vi "利用74HC74设计2-4分频器.vi"() -> ()   [LabVIEW 2018]
panel:
  in  "结束":bool
  out "Q2":bool
  out "Q1":bool
  in  "cp":bool
  # "74HC74：双上升沿D触发器"
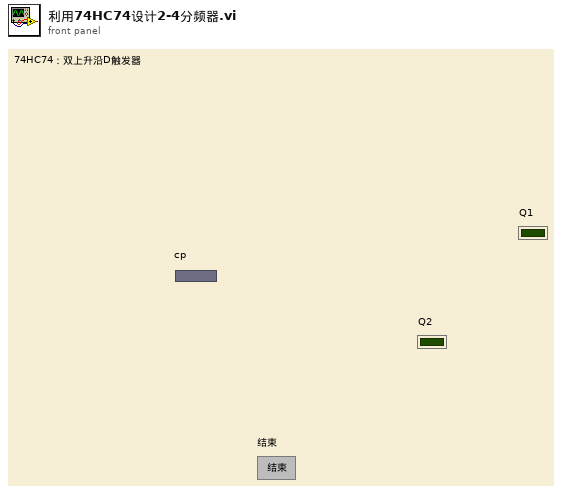
[diagram p1: front panel]
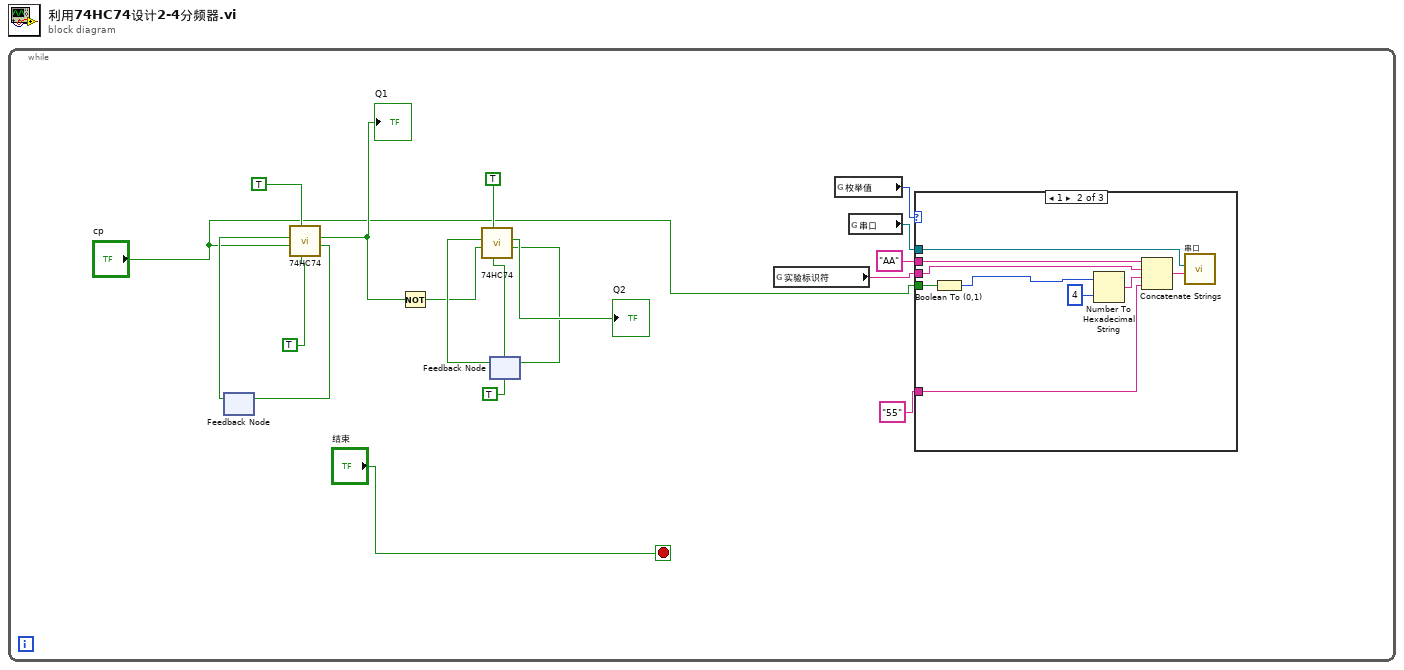
[diagram p0: block diagram]
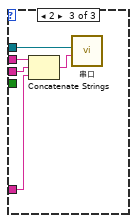
[diagram p3: hidden frame]
diagram:
  n1 = while {
    stop <- "结束" stop-if-true
    n2 = feedback #1() -> (w15:bool)  [unwired: 1 in]
    n3 = call "74HC74.vi"("R`"=TRUE, "S`"=TRUE, "cp"="cp", "D"=w15) -> ("Q`"=w16:bool, "Q"=w8:bool)  [unwired: 6 in]
    "Q1" <- w8
    n4 = feedback-in #1(w16) -> ()
    n5 = Not(x=w8) -> (.not. x?=w9:bool)
    n6 = feedback #2() -> (w10:bool)  [unwired: 1 in]
    n7 = call "74HC74.vi"("R`"=TRUE, "S`"=TRUE, "cp"=w9, "D"=w10) -> ("Q`"=w11:bool, "Q"=→"Q2":bool)  [unwired: 6 in]
    n8 = feedback-in #2(w11) -> ()
    n9 = global read "全局变量.vi" "实验标识符"() -> (w4:string)
    n10 = global read "全局变量.vi" "枚举值"() -> (w6:i8)
    n11 = global read "全局变量.vi" "串口"() -> (w5:refnum<visa-resource-name>)
    n12 = case shown="1" w6 {
      tunnel: "cp" -> [_ w26 _]
      tunnel: w5 -> [_ w25 w30]
      tunnel: w4 -> [_ w24 w31]
      tunnel: "55" -> [_ w23 w28]
      tunnel: "AA" -> [_ w22 w29]
      frame 0, Default {
      }
      frame 1 {
        n13 = Boolean To (0,1)(Boolean=w26) -> (0, 1=w19:i16)
        n14 = Number To Hexadecimal String(1:4, 2:w19) -> (0:w20:string)
        n15 = Concatenate Strings(w22, w24, w20, w23) -> (w27:string)
        n16 = call "串口.vi"("字符串"=w27, "VISA resource name"=w25) -> ()  [unwired: 10 in]
      }
      frame 2 {
        n17 = Concatenate Strings(w29, w31, w28) -> (w32:string)
        n18 = call "串口.vi"("字符串"=w32, "VISA resource name"=w30) -> ()  [unwired: 10 in]
      }
    }
  }
